vi "一个U16转换为double.vi"(10 "低16位_1":u16, 11 "高16位_1":u16) -> (1 "反馈值":dbl)   [LabVIEW 2010]
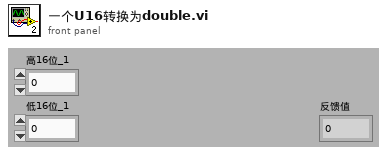
[diagram p1: front panel]
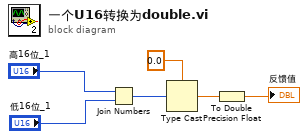
[diagram p0: block diagram]
diagram:
  n1 = Join Numbers(hi="高16位_1", lo="低16位_1") -> ((hi.lo)=w3:u32)
  n2 = Type Cast(type=sgl 0.0, x=w3) -> (*(type *) &x=w2:sgl)
  n3 = To Double Precision Float(number=w2) -> (double precision float=→"反馈值":dbl)
